vi "Broken Rotor Bar Harmonics (N Motors).vi"(0 "spectrum information":T2, 1 "fundamental frequency [Hz]":dbl=50.0, 5 "slip":dbl[](array[numeric]), 7 "max sideband order (10)":u8=10, 11 "error in (no error)":errorcluster) -> (4 "upper sidebands":T1(array[cluster]), 6 "lower sidebands":T1(array[cluster]), 8 "max sideband magnitude [dB]":dbl[](array[numeric]), 15 "error out":errorcluster)   [LabVIEW 2014, in "NI_EP_Motor Monitoring.lvlib"]
doc: "Calculates the sideband harmonics to detect broken rotor bars. You must manually select the polymorphic instance you want to use."
uses:
  <vilib>/addons/Electrical Power/Motor Monitoring/NI_EP_Motor Monitoring.lvlib
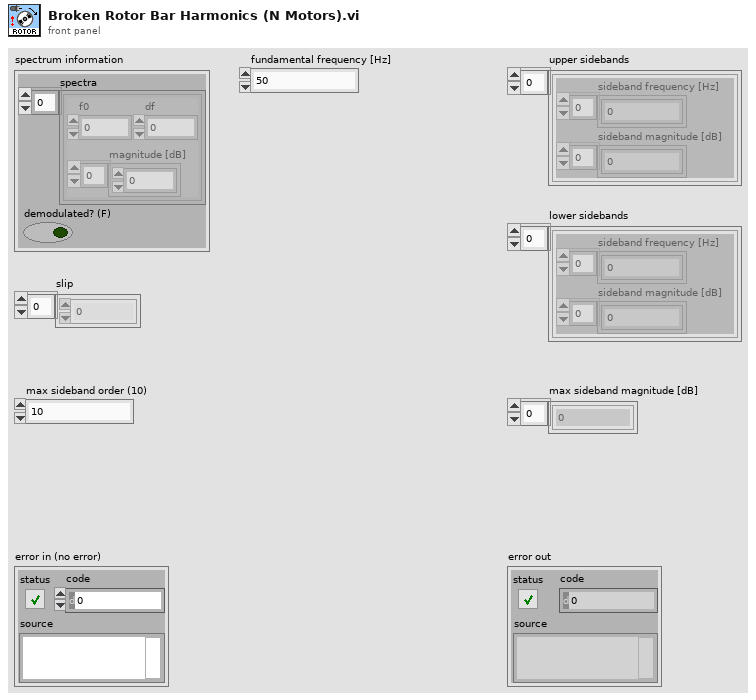
[diagram p1: front panel]
types:
  T1 = cluster{"sideband frequency [Hz]":dbl[], "sideband magnitude [dB]":dbl[]}[]
  T2 = cluster{"spectra":cluster{"f0":dbl, "df":dbl, "magnitude [dB]":dbl[]}[], "demodulated? (F)":bool}
  T3 = cluster{"frequency [Hz]":dbl[], "magnitude [dB]":dbl[]}[]
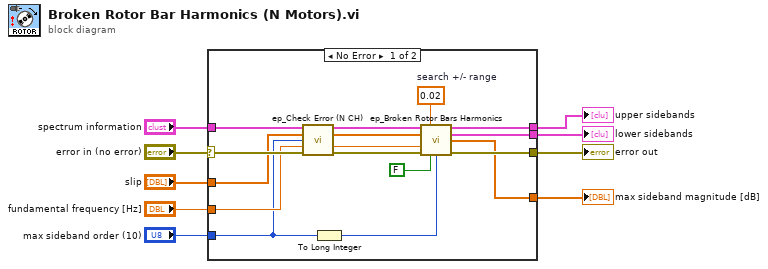
[diagram p0: block diagram]
diagram:
  n1 = case shown="No Error" "error in (no error)" {
    selector: "error in (no error)" -> [w24 w26]
    tunnel: "spectrum information" -> [w22 _]
    tunnel: "fundamental frequency [Hz]" -> [w19 _]
    tunnel: [w25 w26] -> w6
    tunnel: [w21 _] -> w5
    tunnel: [w20 _] -> w4
    tunnel: "slip" -> [w15 _]
    tunnel: "max sideband order (10)" -> [w10 _]
    tunnel: [w13 _] -> w1
    frame No Error {
      w12 = 0.02  # search +/- range
      n2 = call <vilib>:"ep_Check Error (N CH).vi"("spectra information"=w22, "slip"=w15, "max sideband order (10)"=w10, "fundamental frequency [Hz]"=w19, "error in (no error)"=w24) -> ("dup spectra information"=w16:T2, "dup slip"=w18:dbl[], "dup fundamental frequency [Hz]"=w17:dbl, "error out"=w23:errorcluster)  [unwired: 7 in]
      n3 = To Long Integer(number=w10) -> (32bit integer=w14:i32)
      n4 = call <vilib>:"ep_Broken Rotor Bars Harmonics.vi"("spectra information"=w16, "search +/- percentage"=w12, "slip"=w18, "fundamental frequency [Hz]"=w17, "error in (no error)"=w23, "sinc interpolation? (F)"=FALSE, "max sideband order"=w14) -> ("upper sidebands"=w21:T3, "lower sidebands"=w20:T3, "max sideband magnitude [dB]"=w13:dbl[], "error out"=w25:errorcluster)  [unwired: 5 in]
    }
    frame Error {
    }
  }
  "error out" <- w6
  "upper sidebands" <- w5
  "lower sidebands" <- w4
  "max sideband magnitude [dB]" <- w1
